vi "demo - 副本.vi"() -> ()   [LabVIEW 2019]
panel:
  out "Image":T1(plugin-control)
  in  "停止":bool
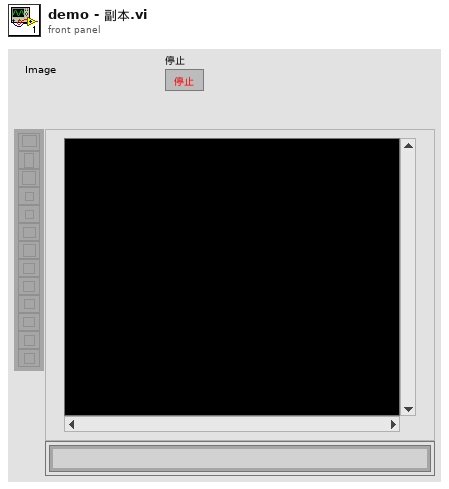
[diagram p1: front panel]
types:
  T1 = typedef "IMAQ Image.ctl" = refnum<image>
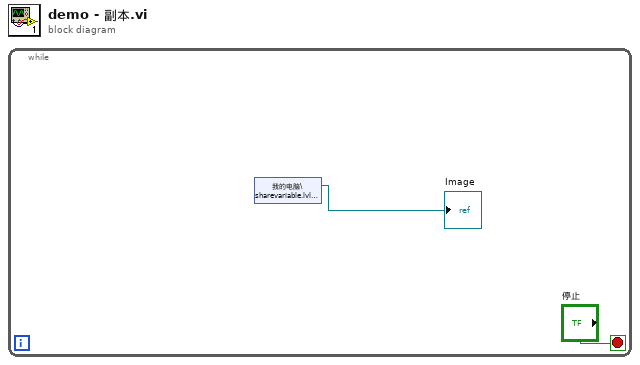
[diagram p0: block diagram]
diagram:
  n1 = while {
    stop <- "停止" stop-if-true
    n2 = shared-variable "我的电脑\\sharevariable.lvlib\\img"() -> (→"Image":refnum<image>)  [unwired: 1 in, 1 out]
  }
